vi "chart series set labels position.vi"(8 "error in (no error)":errorcluster, 10 "position":u8, 11 "series":u32) -> (0 "error out":errorcluster)   [LabVIEW 8.6]
doc: "void chart_series_set_labels_position(lxw_chart_series series, uint8_t position);"
uses:
  pending_lvxlsxwriter/xlsxwriter.dll
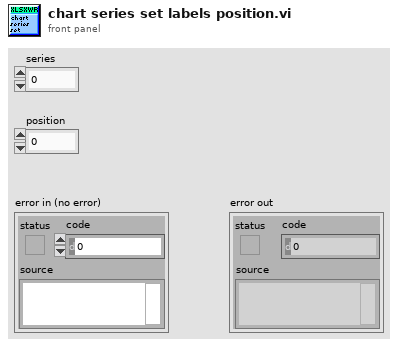
[diagram p1: front panel]
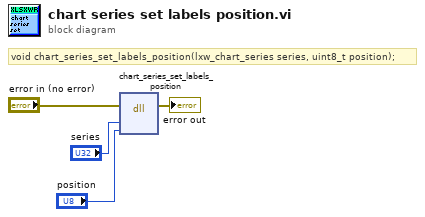
[diagram p0: block diagram]
diagram:
  # "void chart_series_set_labels_position(lxw_chart_series series, uint8_t position);"
  n1 = dll-call lib="C:/Users/WDAGUtilityAccount/Desktop/pending_lvxlsxwriter/xlsxwriter.*" fn="chart_series_set_labels_position"(error in="error in (no error)", "series"="series", "position"="position") -> (error out=→"error out":errorcluster)  [unwired: 5 in, 1 out]
